vi "TEC.vi"() -> ()   [LabVIEW 2025]
panel:
  out "TED":waveform(dbl)[](graph)=[{"t0"=timestamp(3845871052.1406174 s since 1904-01-01), "dt"=1.0, "Y"=[23.85494], "attributes"=variant("NI_ChannelName"=variant(string "TED_Temp_0"))}, {"t0"=timestamp(3845871052.1406174 s since 1904-01-01), "dt"=1.0, "Y"=[0.0], "attributes"=variant("NI_ChannelName"=variant(string "TED_Voltage_0"))}, {"t0"=timestamp(3845871052.1406174 s since 1904-01-01), "dt"=1.0, "Y"=[0.001787742], "attributes"=variant("NI_ChannelName"=variant(string "TED_Current_0"))}, {"t0"=timestamp(3845871052.1406174 s since 1904-01-01), "dt"=1.0, "Y"=[21.97219], "attributes"=variant("NI_ChannelName"=variant(string "TED_Temp_1"))}, {"t0"=timestamp(3845871052.1406174 s since 1904-01-01), "dt"=1.0, "Y"=[0.0], "attributes"=variant("NI_ChannelName"=variant(string "TED_Voltage_1"))}, {"t0"=timestamp(3845871052.1406174 s since 1904-01-01), "dt"=1.0, "Y"=[0.00642528], "attributes"=variant("NI_ChannelName"=variant(string "TED_Current_1"))}]
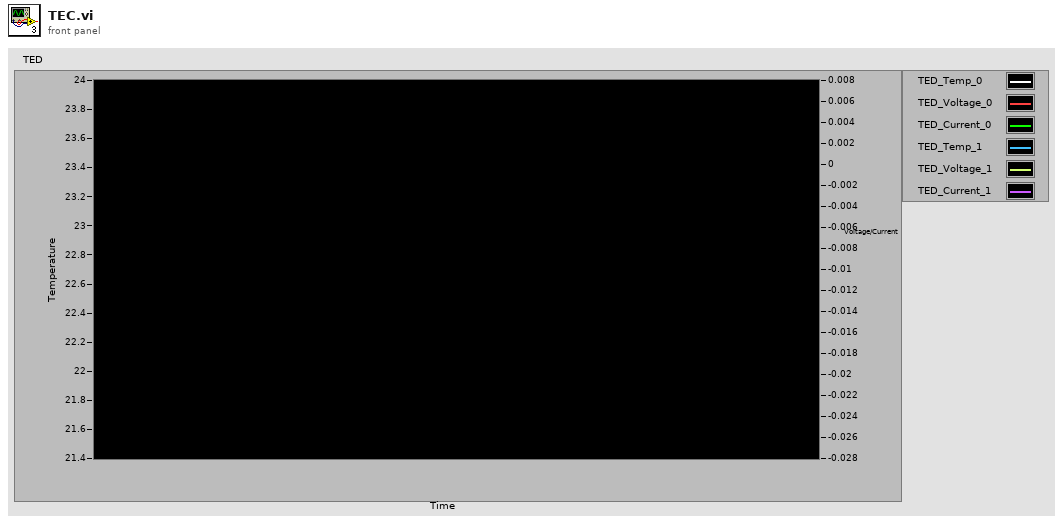
[diagram p1: front panel]
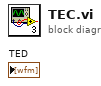
[diagram p0: block diagram]
diagram:
